vi "Save State As Default.vi"(8 "Error In":errorcluster, 11 "Target VI":refnum<vi>) -> (0 "Error Out":errorcluster, 3 "Target VI":refnum<vi>)   [LabVIEW 2011, in "LMH-Toolbox.lvlib"]
uses:
  LMH-Toolbox.lvlib
  Private/VI Tools/LMH-VITools.lvlib
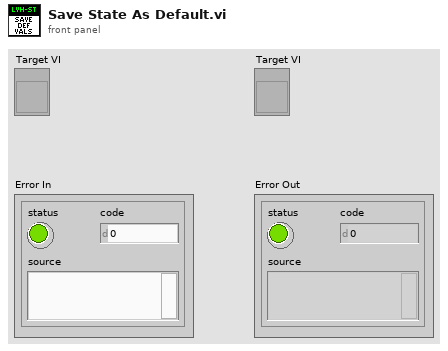
[diagram p1: front panel]
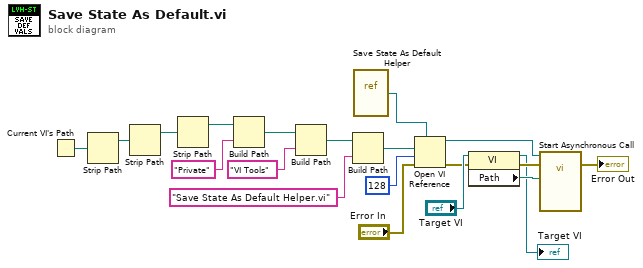
[diagram p0: block diagram]
diagram:
  n1 = Current VI's Path() -> (path=w19:path)
  n2 = Strip Path(path=w19) -> (stripped path=w18:path)  [unwired: 1 out]
  n3 = Strip Path(path=w18) -> (stripped path=w17:path)  [unwired: 1 out]
  n4 = Strip Path(path=w17) -> (stripped path=w16:path)  [unwired: 1 out]
  n5 = Build Path(base path=w16, name or relative path="Private") -> (appended path=w14:path)
  n6 = Build Path(base path=w14, name or relative path="VI Tools") -> (appended path=w11:path)
  n7 = Build Path(base path=w11, name or relative path="Save State As Default Helper.vi") -> (appended path=w10:path)
  n8 = vi-ref "Save State As Default Helper.vi"() -> (w20:refnum<vi>)
  n9 = Open VI Reference(type specifier VI Refnum (for type only)=w20, vi path=w10, options=128, error in (no error)="Error In") -> (vi reference=w9:refnum<vi>, error out=w5:errorcluster)  [unwired: 2 in]
  n10 = property class="VI"(reference="Target VI", error in=w5) -> (reference out=→"Target VI":refnum<vi>, error out=w3:errorcluster, "Path"=w4:path)
  n11 = call-by-ref "Start Asynchronous Call"(reference=w9, error in=w3, "Target VI"=w4) -> (error out=→"Error Out":errorcluster)  [unwired: 10 in, 2 out]
